vi "RSZVB Set RF Off Behavior.vi"(8 "error in (no error)":errorcluster {"code" format="%.0x"}, 9 "RF Off Behavior (Fast)":i32(ring) items=["Fast", "Slow (Lower Broadband Noise)"], 11 "VISA session":refnum<visa-resource-name>) -> (0 "error out":errorcluster {"code" format="%.0x"}, 3 "dup VISA session":refnum<visa-resource-name>)   [LabVIEW 2011]
doc: "This VI configures the behavior of the RF Off switches.\n\nRemote-control command(s):\nOUTPut<1...2>[:STATe]:TYPE"
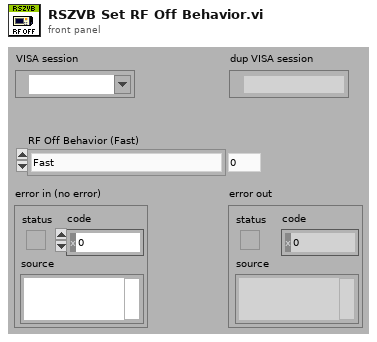
[diagram p1: front panel]
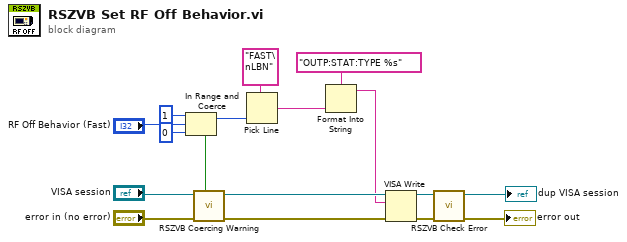
[diagram p0: block diagram]
diagram:
  n1 = In Range and Coerce(upper limit=1 ("lower limit"), x="RF Off Behavior (Fast)", lower limit=0) -> (coerced(x)=w10:i32, In Range?=w12:bool)
  n2 = call "RSZVB Coercing Warning.vi"("In Range?"=w12, "error in (no error)"="error in (no error)", "VISA session"="VISA session") -> ("error out"=w8:errorcluster, "dup VISA session"=w9:refnum<visa-resource-name>)  [unwired: 7 in]
  n3 = Pick Line(multi-line string="FAST\nLBN", line index=w10) -> (output string=w13:string)  [unwired: 1 in]
  n4 = Format Into String(format string="OUTP:STAT:TYPE %s", w13) -> (resulting string=w7:string)  [unwired: 2 in, 1 out]
  n5 = VISA Write(VISA resource name=w9, write buffer=w7, error in (no error)=w8) -> (VISA resource name out=w14:refnum<visa-resource-name>, error out=w15:errorcluster)  [unwired: 1 out]
  n6 = call "RSZVB Check Error.vi"("error in (no error)"=w15, "VISA session"=w14) -> ("error out"=→"error out":errorcluster, "dup VISA session"=→"dup VISA session":refnum<visa-resource-name>)  [unwired: 8 in]
